vi "Reference Provider.vi"() -> (3 "References":T1(array[cluster]))   [LabVIEW 2019]
panel:
  in  "Ring 3":u16(ring) items=["Test Helper 1", "Test Helper 2", "Test Helper 3", "None"]
  in  "Ring 2":u16(ring) items=["Test Helper 1", "Test Helper 2", "Test Helper 3", "None"]
  in  "Ring":u16(ring) items=["Test Helper 1", "Test Helper 2", "Test Helper 3", "None"]
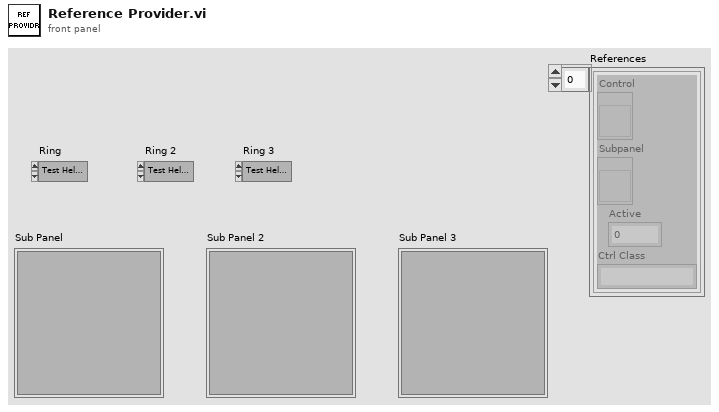
[diagram p1: front panel]
types:
  T1 = cluster{"Control":refnum<vi>, "Subpanel":refnum<vi>, "Active":i32, "Ctrl Class":string}[]
  T2 = cluster{"Control":refnum<vi>, "Subpanel":refnum<vi>, "Active":i32, "Ctrl Class":string}
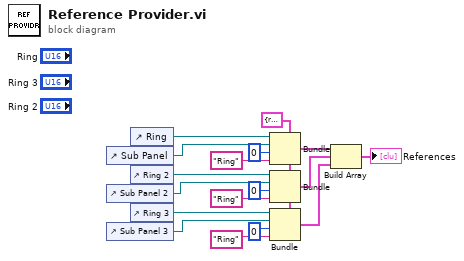
[diagram p0: block diagram]
diagram:
  w11 = T2 {"Control"=refnum, "Subpanel"=refnum, "Active"=0, "Ctrl Class"=""} ("Panel")
  n1 = control-ref of="Sub Panel"() -> (w16:refnum<vi>)
  n2 = control-ref of="Sub Panel 2"() -> (w14:refnum<vi>)
  n3 = control-ref of="Sub Panel 3"() -> (w12:refnum<vi>)
  n4 = control-ref of="Ring"() -> (w17:refnum<vi>)
  n5 = control-ref of="Ring 2"() -> (w15:refnum<vi>)
  n6 = control-ref of="Ring 3"() -> (w13:refnum<vi>)
  n7 = Bundle(cluster=w11, "Control"=w17, "Subpanel"=w16, "Active"=0, "Ctrl Class"="Ring") -> (w4:T2)
  n8 = Bundle(cluster=w11, "Control"=w15, "Subpanel"=w14, "Active"=0, "Ctrl Class"="Ring") -> (w3:T2)
  n9 = Bundle(cluster=w11, "Control"=w13, "Subpanel"=w12, "Active"=0, "Ctrl Class"="Ring") -> (w2:T2)
  n10 = Build Array(w4, w3, w2) -> (→"References":T1)
